vi "Get Active Timing Function.vi"(0 "Timing Functions in":refnum<class "Timing Functions.lvclass">, 11 "error in (no error)":errorcluster) -> (4 "Timing Functions out":refnum<class "Timing Functions.lvclass">, 6 "Function List":T1, 15 "error out":errorcluster)   [LabVIEW 2016, in "Timing Functions.lvclass"]
uses:
  Timing Functions.lvclass
  E:/Repository/LabVIEW Script Language/source code/LSL components/functions/functionsbase/functionbase.lvclass
  Function List.ctl
  functionsbase/functionbase.lvclass
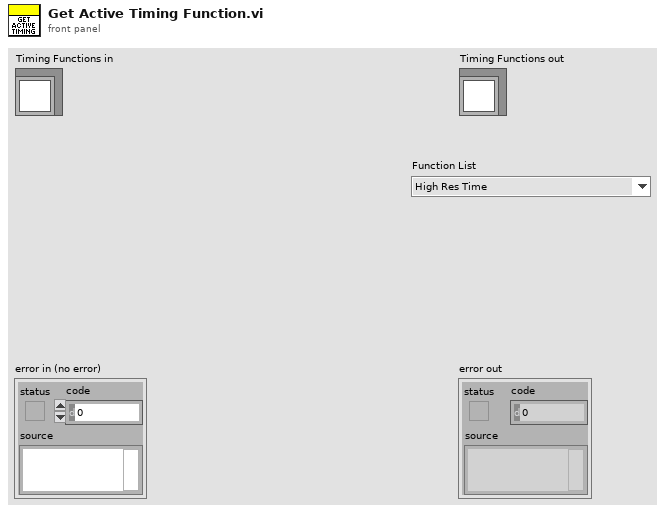
[diagram p1: front panel]
types:
  T1 = typedef "Timing Functions.lvclass/Function List.ctl" = enum16{"High Res Time", "Wait", "Get Date and Time"}
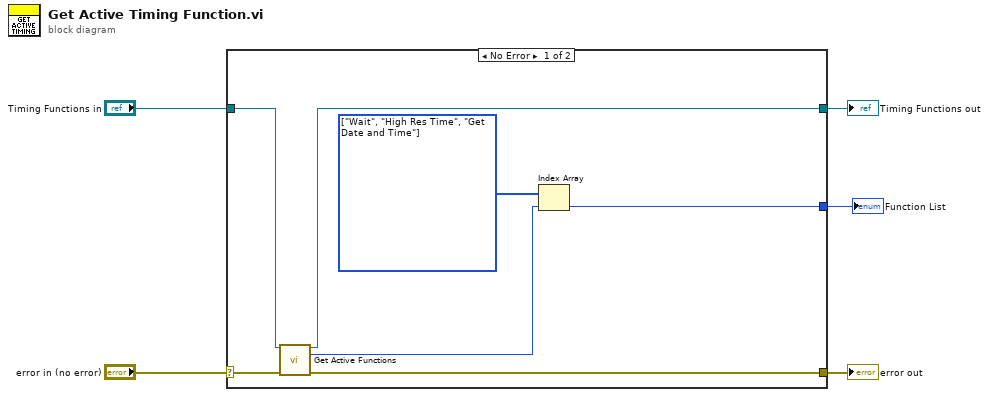
[diagram p0: block diagram]
diagram:
  n1 = case shown="No Error" "error in (no error)" {
    selector: "error in (no error)" -> [w12 w14]
    tunnel: [w11 w14] -> w4
    tunnel: [w9 w13] -> w2
    tunnel: "Timing Functions in" -> [w10 w13]
    tunnel: [w6 _] -> w1
    frame No Error {
      w8 = T1[] [enum."Wait", enum."High Res Time", enum."Get Date and Time"] items=["High Res Time", "Wait", "Get Date and Time"]
      n2 = call "Get Active Functions.vi"("functionbase in"=w10, "error in (no error)"=w12) -> ("functionbase out"=w9:refnum<class "Timing Functions.lvclass">, "Syntax Index"=w7:i32, "error out"=w11:errorcluster)  [unwired: 11 in]
      n3 = Index Array(array=w8, index=w7) -> (element=w6:T1)
    }
    frame Error {
    }
  }
  "error out" <- w4
  "Timing Functions out" <- w2
  "Function List" <- w1
